vi "LVJSON Find.vi"(10 "Key":string, 11 "Elements in":T1[](array[typedef])) -> (2 "Found?":bool, 3 "Index":i32)   [LabVIEW 2018, in "labview_json.lvlib"]
uses:
  labview_json.lvlib
  Element Type.ctl
  Element.ctl
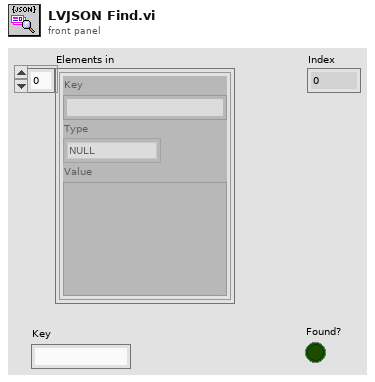
[diagram p1: front panel]
types:
  T1 = typedef "labview_json.lvlib/Element.ctl" = cluster{"Key":string, "Type":T2, "Value":variant}
  T2 = typedef "labview_json.lvlib/Element Type.ctl" = enum8{"NULL", "BOOL", "INT", "UINT", "FLOAT", "STRING", "ARRAY", "OBJECT", "SKIP"}
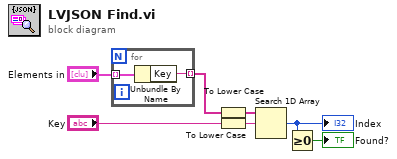
[diagram p0: block diagram]
diagram:
  n1 = for {
    tunnel: "Elements in" -> [w9] mode=indexing
    tunnel: [w8] -> w7 mode=indexing
    n2 = Unbundle By Name(w9) -> ("Key"=w8:string)
  }
  n3 = To Lower Case(string=w7) -> (all lower case string=w5:string[])
  n4 = To Lower Case(string="Key") -> (all lower case string=w4:string)
  n5 = Search 1D Array(1D array=w5, element=w4) -> (index of element=w2:i32)  [unwired: 1 in]
  "Index" <- w2
  n6 = Greater Or Equal To 0?(x=w2) -> (x >= 0?=→"Found?":bool)
